vi "read_csv_v01.vi"() -> ()   [LabVIEW 2024]
uses:
  <vilib>/Utility/file.llb/Read Delimited Spreadsheet (string).vi
panel:
  out "元素 2":string
  out "元素":string
  out "数组":string[](array[string])
  out "all rows":string[][](array[string]) caption="所有行"
  out "测试脚本配置输出":T1(array[cluster])
  in  "簇":T2
  out "脚本每行":string[](array[string])
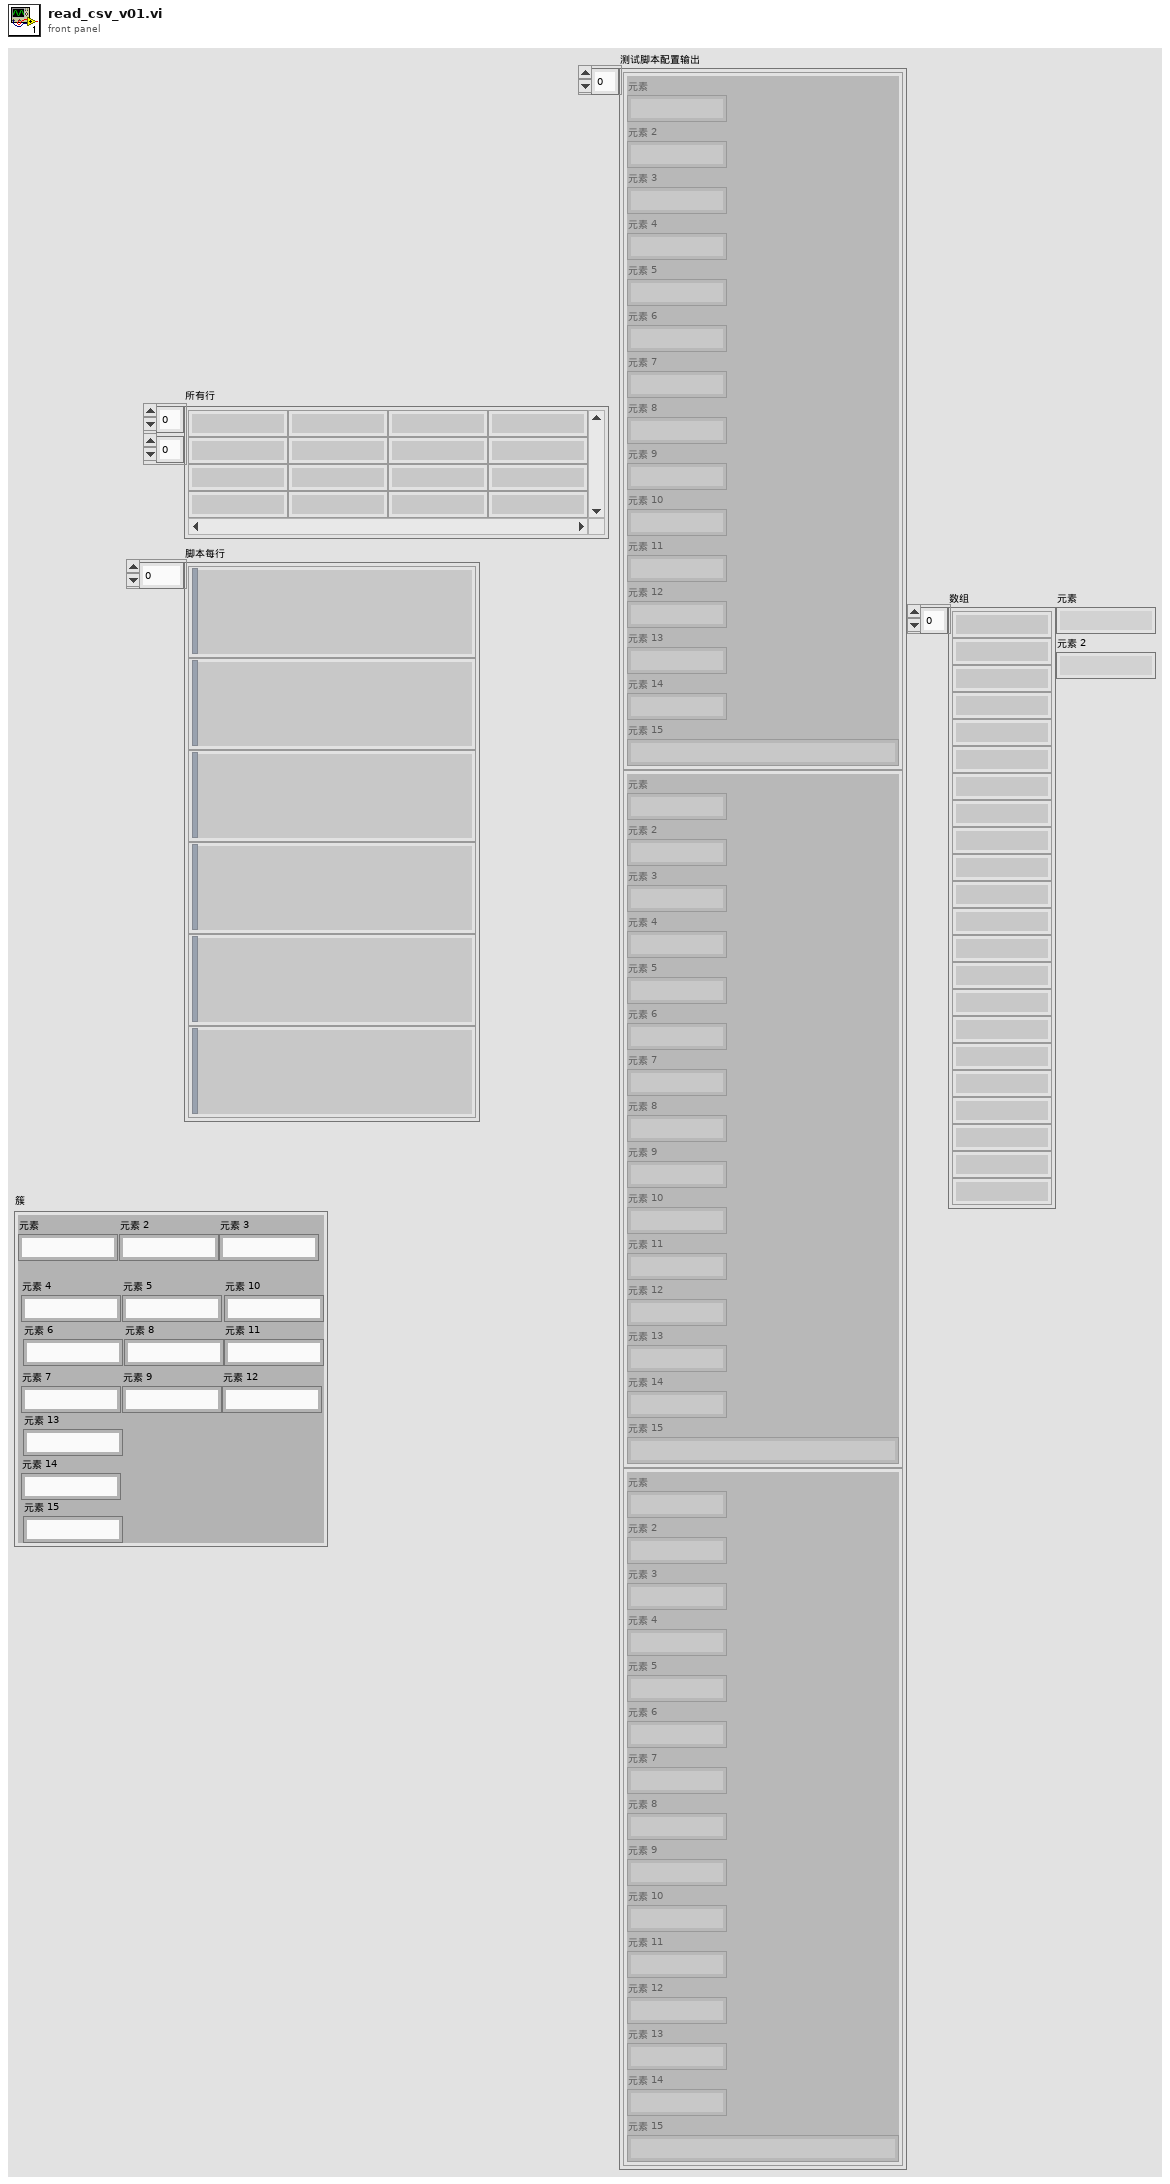
[diagram p1: front panel]
types:
  T1 = cluster{"元素":string, "元素 2":string, "元素 3":string, "元素 4":string, "元素 5":string, "元素 6":string, "元素 7":string, "元素 8":string, "元素 9":string, "元素 10":string, "元素 11":string, "元素 12":string, "元素 13":string, "元素 14":string, "元素 15":string}[]
  T2 = cluster{"元素":string, "元素 2":string, "元素 3":string, "元素 4":string, "元素 5":string, "元素 6":string, "元素 7":string, "元素 8":string, "元素 9":string, "元素 10":string, "元素 11":string, "元素 12":string, "元素 13":string, "元素 14":string, "元素 15":string}
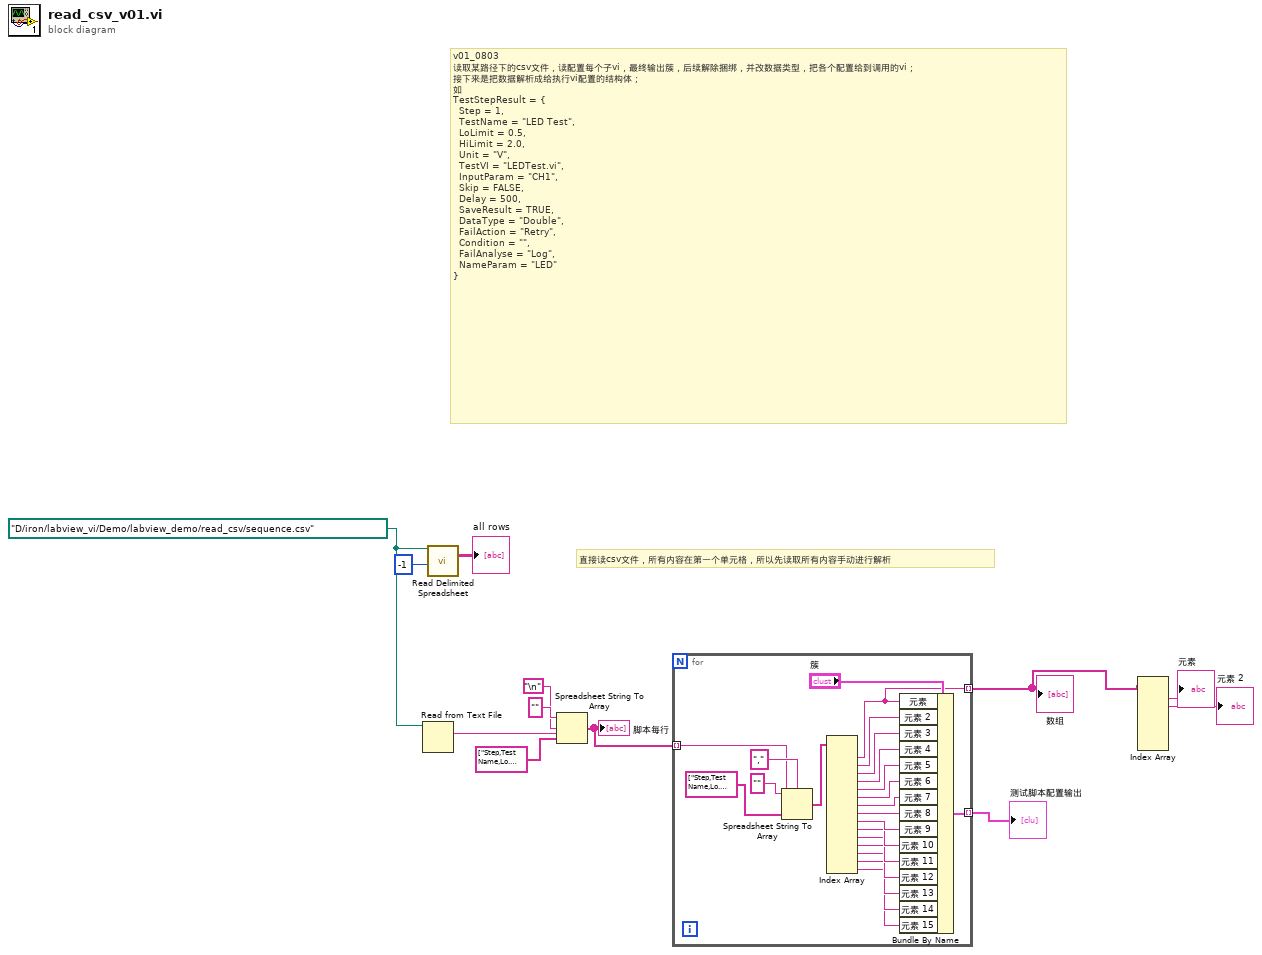
[diagram p0: block diagram]
diagram:
  w5 = path "D:/iron/labview_vi/Demo/labview_demo/read_csv/sequence.csv" ("file path (dialog if empty)")
  # "直接读csv文件，所有内容在第一个单元格，所以先读取所有内容手动进行解析"
  # "v01_0803\n读取某路径下的csv文件，读配置每个子vi，最终输出簇，后续解除捆绑，并改数据类型，把各个配置给到调用的vi；\n接下来是把数据解析成给执行vi配置的结构体；\n如\nTestStepResult = {\n  Step = 1,\n  TestName = \"LED Test\",\n  LoLimit = 0.5,\n  HiLimit = 2.0,\n  Unit = \"V\",\n  TestVI = \"LEDTest.vi\",\n  InputParam = \"CH1\",\n  Skip = FALSE,\n  Delay = 500,\n  SaveResult = TRUE,\n  DataType = \"Double\",\n  FailAction = \"Retry\",\n  Condition = \"\",\n  FailAnalyse = \"Log\",\n  NameParam = \"LED\"\n}"
  n1 = Read from Text File(file (use dialog)=w5) -> (text=w11:string)  [unwired: 3 in, 3 out]
  n2 = call-poly <vilib>:"Read Delimited Spreadsheet.vi"("file path (dialog if empty)"=w5, "number of rows (all:-1)"=-1) -> ("all rows"=→"all rows":string[][])  [unwired: 8 in, 5 out]
  n3 = Spreadsheet String To Array(delimiter (Tab)="\n", format string="" ("格式字符串"), spreadsheet string=w11, array type (2D Dbl)=string[] ["Step,Test Name,Lo.Limit,Hi.Limit,Unit,Test Vi Name,Input Parameter,Skip,Delay,Save Result,Data Type,Fail Action,Condition,Fail Analyse,Name Parameter"] ("添加的数组")) -> (array=w7:string[])
  "脚本每行" <- w7
  n4 = for {
    tunnel: w7 -> [w31] mode=indexing
    tunnel: [w29] -> w6 mode=indexing
    tunnel: [w13] -> w3 mode=indexing
    n5 = Spreadsheet String To Array(delimiter (Tab)="," ("正则表达式"), format string="" ("格式字符串"), spreadsheet string=w31, array type (2D Dbl)=string[] ["Step,Test Name,Lo.Limit,Hi.Limit,Unit,Test Vi Name,Input Parameter,Skip,Delay,Save Result,Data Type,Fail Action,Condition,Fail Analyse,Name Parameter", "1,,,,,,,,,,,,,,", "12,,,,,,,,,,,,,,", ""] ("数组 2")) -> (array=w33:string[])
    n6 = Index Array(array=w33) -> (element #1=w13:string, element #2=w30:string, element #3=w28:string, element #4=w27:string, element #5=w26:string, element #6=w25:string, element #7=w24:string, element #8=w23:string, element #9=w22:string, element #10=w21:string, element #11=w20:string, element #12=w19:string, element #13=w18:string, element #14=w17:string, element #15=w16:string)  [unwired: 15 in]
    n7 = Bundle By Name(cluster="簇", "元素"=w13, "元素 2"=w30, "元素 3"=w28, "元素 4"=w27, "元素 5"=w26, "元素 6"=w25, "元素 7"=w24, "元素 8"=w23, "元素 9"=w22, "元素 10"=w21, "元素 11"=w20, "元素 12"=w19, "元素 13"=w18, "元素 14"=w17, "元素 15"=w16) -> (w29:T2)
  }
  "测试脚本配置输出" <- w6
  "数组" <- w3
  n8 = Index Array(array=w3) -> (element #1=→"元素":string, element #2=→"元素 2":string)  [unwired: 7 in, 5 out]
